vi "Get SMO HELP.vi"(8 "error in (no error)":errorcluster, 10 "Command":string, 11 "Instrument.Lockin in":refnum<class "Instrument.Lockin.lvclass">) -> (0 "error out":errorcluster, 2 "help cluster":T1, 3 "Instrument.Lockin out":refnum<class "Instrument.Lockin.lvclass">)   [LabVIEW 2019, in "Instrument.Lockin.lvlib" / "Instrument.Lockin.lvclass"]
uses:
  Instrument.Lockin.lvclass
  <userlib>/LevyLab/Instrument Framework/subsystems/Help/typedefs/Help--cluster.ctl
  Typedefs/API/Lockin.Commands--Enum.ctl
  Instrument.DAQ/Typedefs/AO.Channel--Cluster.ctl
  Instrument.DAQ/Typedefs/AO.Channel.Function--Enum.ctl
  Instrument.DAQ/Typedefs/AO.Channel--Cluster--Array.ctl
  Typedefs/API/Lockin.setAO_Amp--cluster.ctl
  Typedefs/API/Lockin.setAO_DC--cluster.ctl
  Typedefs/API/Lockin.setAO_f--cluster.ctl
  Typedefs/API/Lockin.setAO_phi--cluster.ctl
  Typedefs/API/Lockin.setAO_function--cluster.ctl
  Instrument.DAQ/Typedefs/REF.Channel--Cluster.ctl
  Instrument.DAQ/Typedefs/REF.Channel--Cluster--Array.ctl
  Typedefs/API/Lockin.setREF_f--cluster.ctl
  Typedefs/API/Lockin.setREF_phi--cluster.ctl
  Typedefs/API/Lockin.setREF_TC--cluster.ctl
  Typedefs/API/Lockin.setREF_RollOff--cluster.ctl
  Instrument.DAQ/Typedefs/DAQ.Configuration--Cluster.ctl
  Instrument.DAQ/Typedefs/DAQ.Config.AO.Range--enum.ctl
  Instrument.DAQ/Typedefs/DAQ.TerminalConfiguration--ring.ctl
  Instrument.DAQ/Typedefs/DAQ.Config.AI.Range--enum.ctl
  Instrument.DAQ/Typedefs/DAQ.Config.AI.Coupling--enum.ctl
  Instrument.DAQ/Typedefs/DAQ.Configuration--Cluster--Array.ctl
  <userlib>/LevyLab/Instrument Framework/Instrument Types/Lockin/Typedefs/LockinAPI.Sampling.Sampling--Cluster.ctl
  Typedefs/API/Lockin.setState--cluster.ctl
  Instrument.DAQ/Typedefs/State--enum.ctl
  Instrument.DAQ/Typedefs/Sweep.Configuration--Cluster.ctl
  Instrument.DAQ/Typedefs/Sweep.Channel--Cluster--Array.ctl
  Instrument.DAQ/Typedefs/Sweep.Channel--Cluster.ctl
  Instrument.DAQ/Typedefs/Sweep.Pattern--Enum.ctl
  Typedefs/API/Lockin.setSweep_Time--cluster.ctl
  Typedefs/API/Lockin.setSweep_Table--cluster.ctl
  <userlib>/LevyLab/Instrument Framework/Instrument Types/Lockin/Typedefs/LockinAPI.getState.states--enum.ctl
  Instrument.DAQ/Typedefs/Results--Cluster.ctl
  <userlib>/LevyLab/Instrument Framework/Instrument Types/Lockin/Typedefs/LockinAPI.SweepData--Cluster.ctl
  <userlib>/LevyLab/Instrument Framework/Instrument Types/Lockin/Instrument.LockinAPI.lvclass
  <userlib>/LevyLab/Instrument Framework/Instrument/Typedefs/Instrument.IDN--cluster.ctl
  <userlib>/LevyLab/Instrument Framework/Instrument/Instrument.lvclass
  <vilib>/PRIrvin/JSON-Schema/JSON-Schema.lvlib
  Instrument.DAQ/Instrument.DAQ.lvclass
  <userlib>/LevyLab/Instrument Framework/subsystems/Help/Help.lvclass
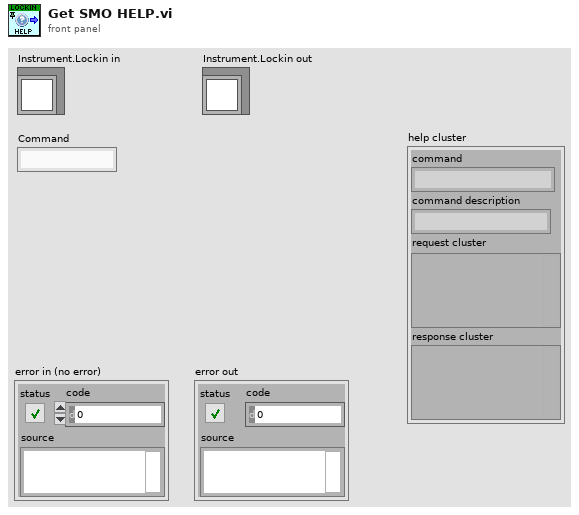
[diagram p1: front panel]
types:
  T1 = typedef "Instrument.lvlib/Help.lvclass/Help--cluster.ctl" = cluster{"command":string, "command description":string, "request cluster":variant, "response cluster":variant}
  T2 = typedef "Instrument.Lockin.lvlib/Instrument.Lockin.lvclass/Lockin.Commands--Enum.ctl" = enum16{"setAO", "setAO_Amplitude", "setAO_DC", "setAO_Frequency", "setAO_Phase", "setAO_Function", "setREF", "setREF_Frequency", "setREF_Phase", "setREF_TC", "setREF_Roll-Off", "setDAQ", "setSampling", "setState", "getState", "getAO", "getAI", "getResults", "getSampling", "getAOconfig", "getREFconfig", "setInputGain", "setOutputGain", "getInputGain", "getOutputGain", "setSweep", "setSweep_Time", "setSweep_Table", "getStatus", "getSweepResults", "getSweepWaveforms", "logConfiguration", "startLogging", "stopLogging"}
  T3 = typedef "Instrument.Lockin.lvlib/Instrument.DAQ.lvclass/AO.Channel--Cluster.ctl" = cluster{"Enable?":bool, "Channel":i32, "Amplitude":dbl, "Offset":dbl, "Frequency":dbl, "Phase":dbl, "Function":T4, "Sweeping?":bool, "Limit AC":bool, "Limit DC?":bool, "Duty Cycle":bool}
  T4 = typedef "Instrument.Lockin.lvlib/Instrument.DAQ.lvclass/AO.Channel.Function--Enum.ctl" = enum16{"sine", "square", "triangle", "saw"}
  T5 = typedef "Instrument.Lockin.lvlib/Instrument.DAQ.lvclass/REF.Channel--Cluster.ctl" = cluster{"Enable?":bool, "Channel":i32, "Frequency":dbl, "Phase":dbl, "TC":dbl, "Roll-Off":i32}
  T6 = typedef "Instrument.Lockin.lvlib/Instrument.DAQ.lvclass/DAQ.Configuration--Cluster.ctl" = cluster{"Device":string, "Lockin.AO":string, "AO.Ch":string, "AO.Range":T7, "AO terminal config":T8, "Lockin.AI":string, "AI.Ch":string, "AI.Range":T9, "AI.Coupling":T10, "AI terminal config":T8}
  T7 = typedef "Instrument.Lockin.lvlib/Instrument.DAQ.lvclass/DAQ.Config.AO.Range--enum.ctl" = enum16{"±0.1", "±1.0", "±3.5", "±10.0", ""}
  T8 = typedef "Instrument.Lockin.lvlib/Instrument.DAQ.lvclass/DAQ.TerminalConfiguration--ring.ctl" = i32
  T9 = typedef "Instrument.Lockin.lvlib/Instrument.DAQ.lvclass/DAQ.Config.AI.Range--enum.ctl" = enum16{"±0.316", "±1.00", "±3.16", "±10.0", "±31.6", "±42.4", ""}
  T10 = typedef "Instrument.Lockin.lvlib/Instrument.DAQ.lvclass/DAQ.Config.AI.Coupling--enum.ctl" = u16
  T11 = typedef "Instrument.Lockin.lvlib/Instrument.Lockin.lvclass/Lockin.setSweep_Table--cluster.ctl" = cluster{"Channel":i32, "Table":dbl[]}
  T12 = typedef "Instrument.LockinAPI.lvclass/LockinAPI.SweepData--Cluster.ctl" = cluster{"AO":waveform(dbl)[], "AI":waveform(dbl)[], "X":waveform(dbl)[], "Y":waveform(dbl)[]}
  T13 = typedef "Instrument.Lockin.lvlib/Instrument.DAQ.lvclass/AO.Channel--Cluster--Array.ctl" = T3[]
  T14 = typedef "Instrument.Lockin.lvlib/Instrument.Lockin.lvclass/Lockin.setAO_Amp--cluster.ctl" = cluster{"Channel":i32, "Amplitude":dbl}
  T15 = typedef "Instrument.Lockin.lvlib/Instrument.Lockin.lvclass/Lockin.setAO_DC--cluster.ctl" = cluster{"Channel":i32, "DC":dbl}
  T16 = typedef "Instrument.Lockin.lvlib/Instrument.Lockin.lvclass/Lockin.setAO_f--cluster.ctl" = cluster{"Channel":i32, "Frequency":dbl}
  T17 = typedef "Instrument.Lockin.lvlib/Instrument.Lockin.lvclass/Lockin.setAO_phi--cluster.ctl" = cluster{"Channel":i32, "Phase":dbl}
  T18 = typedef "Instrument.Lockin.lvlib/Instrument.Lockin.lvclass/Lockin.setAO_function--cluster.ctl" = cluster{"Channel":i32, "Function":T4}
  T19 = typedef "Instrument.Lockin.lvlib/Instrument.DAQ.lvclass/REF.Channel--Cluster--Array.ctl" = T5[]
  T20 = typedef "Instrument.Lockin.lvlib/Instrument.Lockin.lvclass/Lockin.setREF_f--cluster.ctl" = cluster{"Channel":i32, "Frequency":dbl}
  T21 = typedef "Instrument.Lockin.lvlib/Instrument.Lockin.lvclass/Lockin.setREF_phi--cluster.ctl" = cluster{"Channel":i32, "Phase":dbl}
  T22 = typedef "Instrument.Lockin.lvlib/Instrument.Lockin.lvclass/Lockin.setREF_TC--cluster.ctl" = cluster{"Channel":i32, "TC":dbl}
  T23 = typedef "Instrument.Lockin.lvlib/Instrument.Lockin.lvclass/Lockin.setREF_RollOff--cluster.ctl" = cluster{"Channel":i32, "Roll-Off":i32}
  T24 = typedef "Instrument.Lockin.lvlib/Instrument.DAQ.lvclass/DAQ.Configuration--Cluster--Array.ctl" = T6[]
  T25 = typedef "Instrument.LockinAPI.lvclass/LockinAPI.Sampling.Sampling--Cluster.ctl" = cluster{"Fs":dbl, "#s":i32}
  T26 = typedef "Instrument.Lockin.lvlib/Instrument.Lockin.lvclass/Lockin.setState--cluster.ctl" = cluster{"State":T27}
  T27 = typedef "Instrument.Lockin.lvlib/Instrument.DAQ.lvclass/State--enum.ctl" = enum16{"start", "stop", "reset", "start sweep", "stop sweep"}
  T28 = typedef "Instrument.Lockin.lvlib/Instrument.DAQ.lvclass/Sweep.Configuration--Cluster.ctl" = cluster{"sweepTime":dbl, "initialWaitTime":dbl, "returnToStart":bool, "sweepChannels":T29}
  T29 = typedef "Instrument.Lockin.lvlib/Instrument.DAQ.lvclass/Sweep.Channel--Cluster--Array.ctl" = T30[]
  T30 = typedef "Instrument.Lockin.lvlib/Instrument.DAQ.lvclass/Sweep.Channel--Cluster.ctl" = cluster{"Enable?":bool, "Channel":u16, "Start":dbl, "End":dbl, "Pattern":T31, "Table":dbl[]}
  T31 = typedef "Instrument.Lockin.lvlib/Instrument.DAQ.lvclass/Sweep.Pattern--Enum.ctl" = enum16{"Ramp /", "Ramp /\\", "Smooth Ramp _/", "Smooth Ramp _/\\_", "Table"}
  T32 = typedef "Instrument.Lockin.lvlib/Instrument.Lockin.lvclass/Lockin.setSweep_Time--cluster.ctl" = cluster{"SweepTime":dbl}
  T33 = typedef "Instrument.LockinAPI.lvclass/LockinAPI.getState.states--enum.ctl" = enum16{"idle", "created", "started", "stopped", "sweeping"}
  T34 = typedef "Instrument.Lockin.lvlib/Instrument.DAQ.lvclass/Results--Cluster.ctl" = cluster{"Time Stamp":timestamp, "Results (Dictionary)":cluster{"key":string, "value":dbl[]}[]}
  T35 = typedef "Instrument.lvlib/Instrument.lvclass/Instrument.IDN--cluster.ctl" = cluster{"vendor":string, "model":string, "serial":string, "firmware":string}
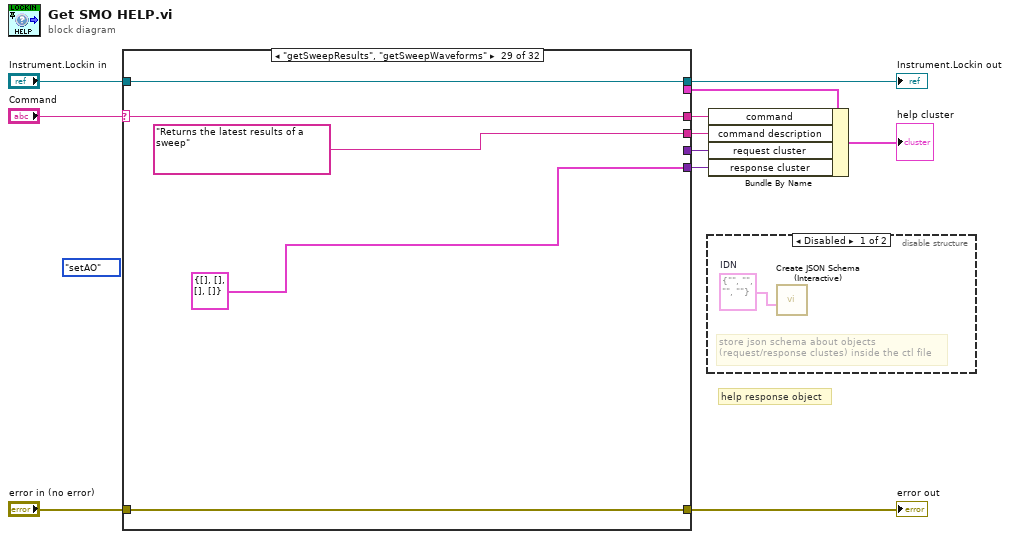
[diagram p0: block diagram]
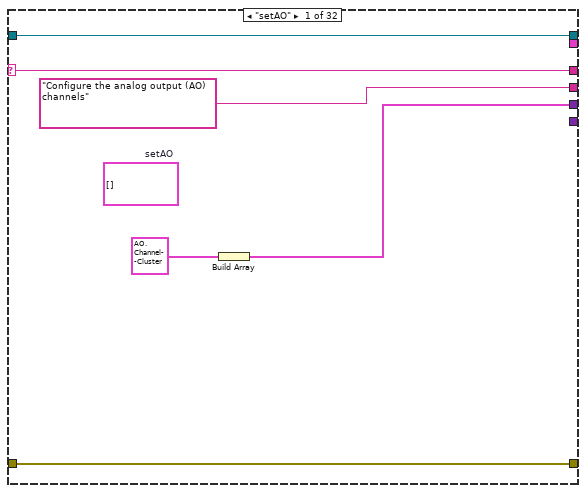
[diagram p2: hidden frame]
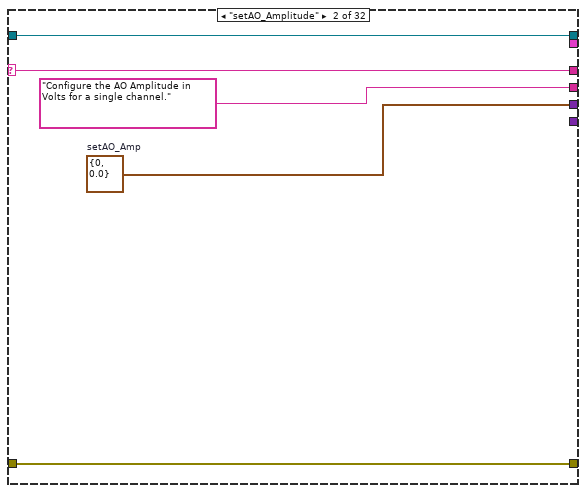
[diagram p3: hidden frame]
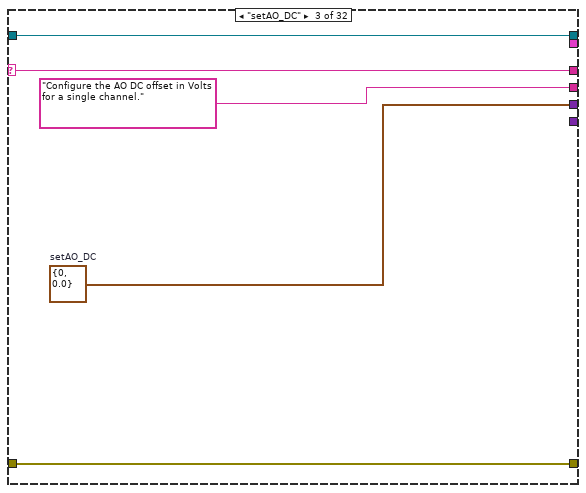
[diagram p4: hidden frame]
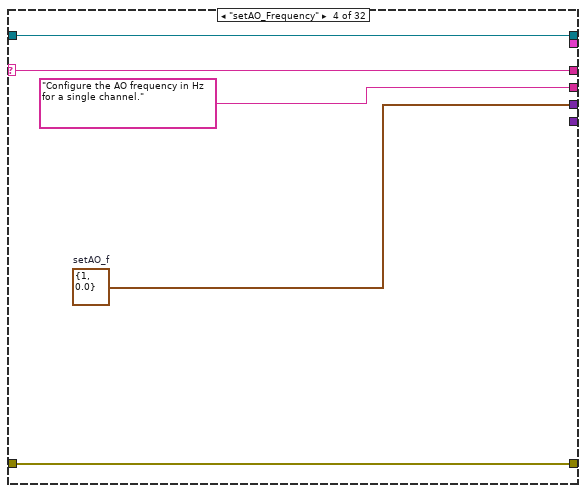
[diagram p5: hidden frame]
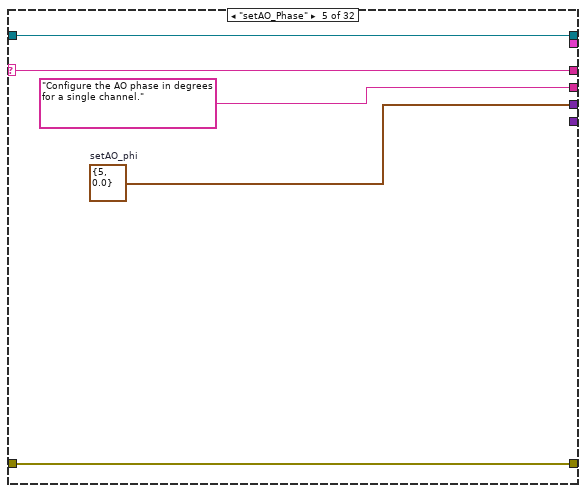
[diagram p6: hidden frame]
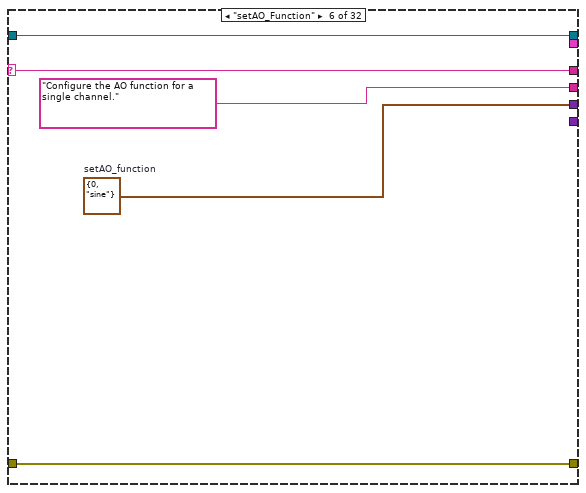
[diagram p7: hidden frame]
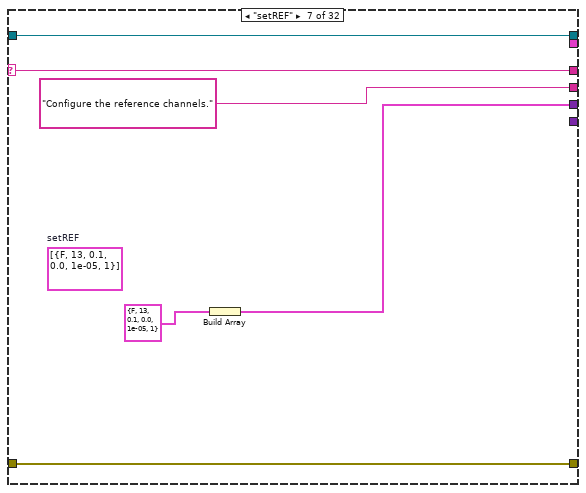
[diagram p8: hidden frame]
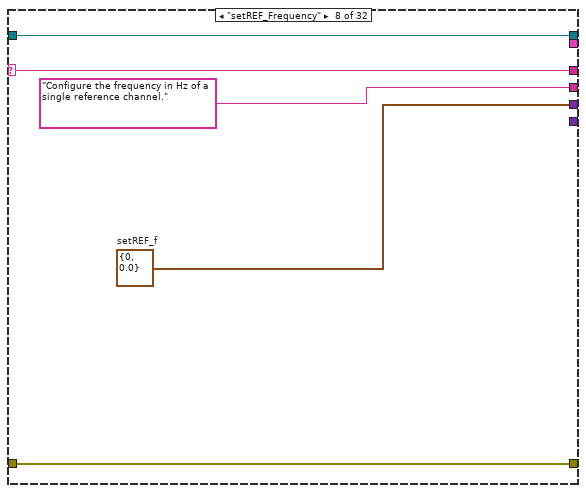
[diagram p9: hidden frame]
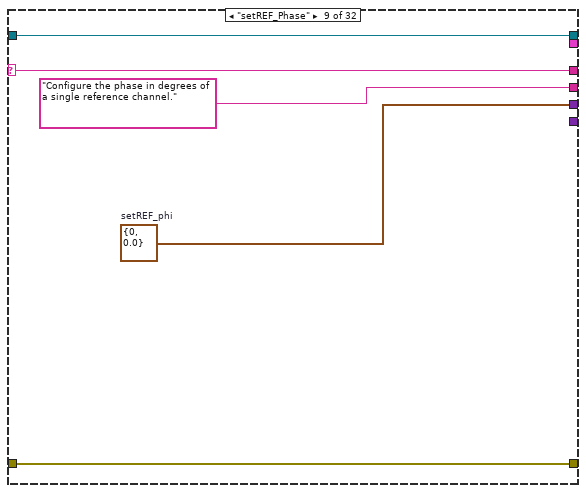
[diagram p10: hidden frame]
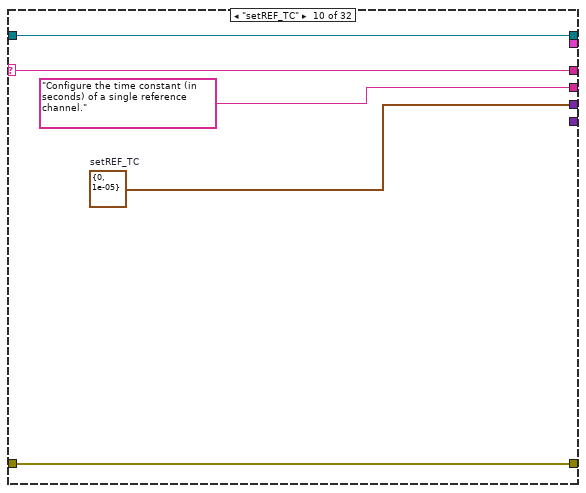
[diagram p11: hidden frame]
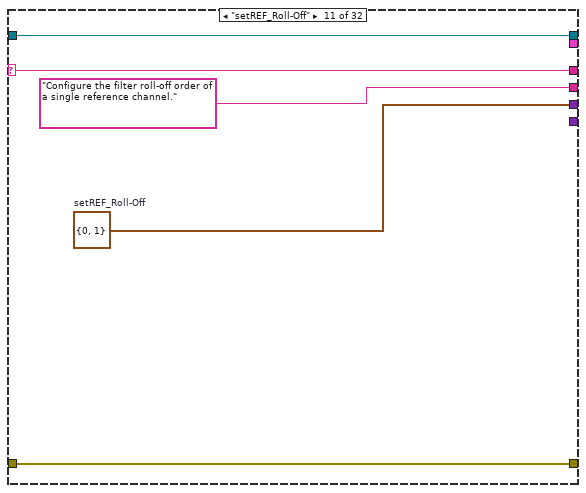
[diagram p12: hidden frame]
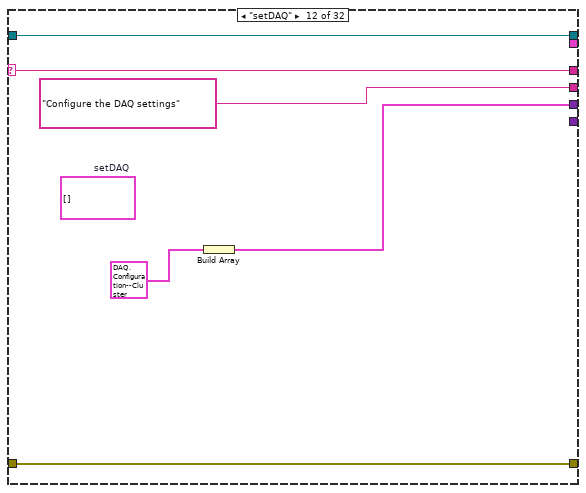
[diagram p13: hidden frame]
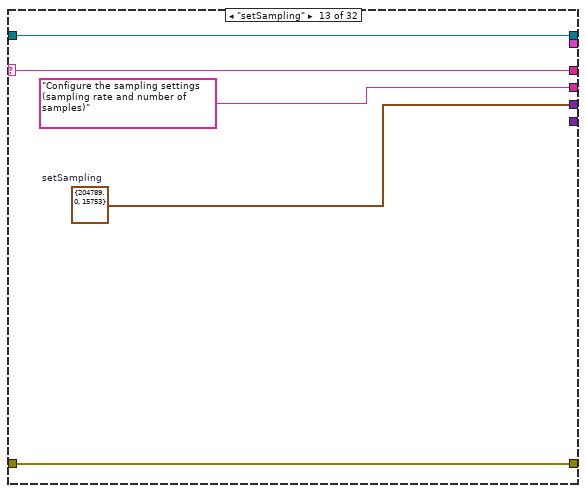
[diagram p14: hidden frame]
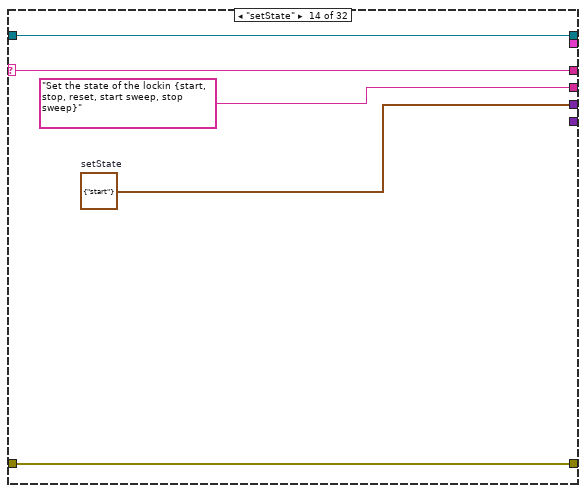
[diagram p15: hidden frame]
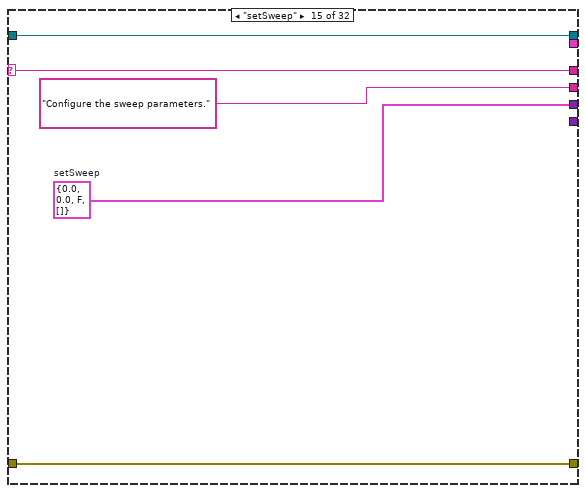
[diagram p16: hidden frame]
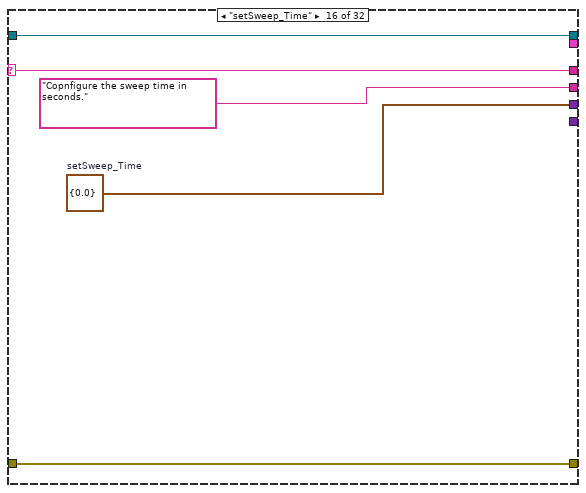
[diagram p17: hidden frame]
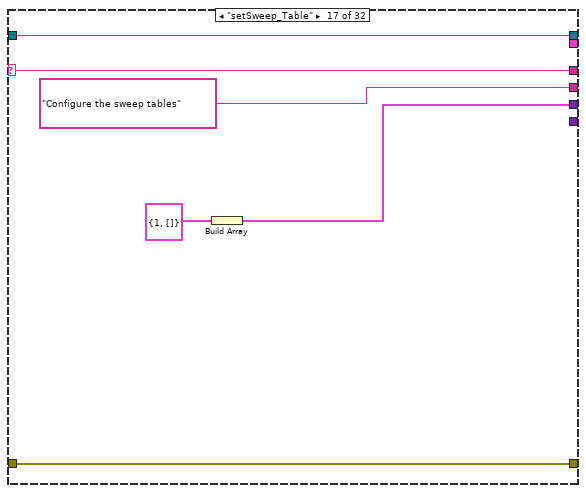
[diagram p18: hidden frame]
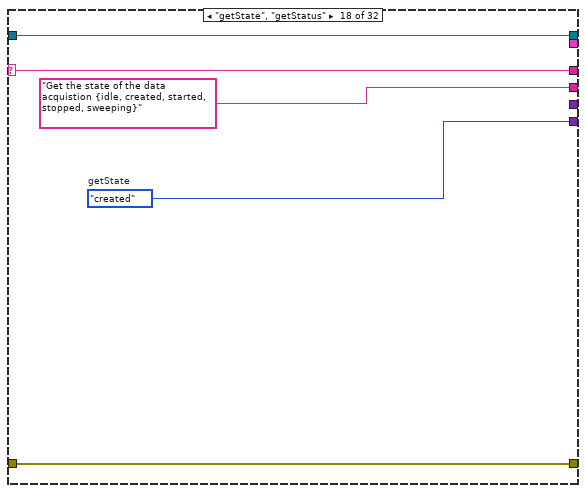
[diagram p19: hidden frame]
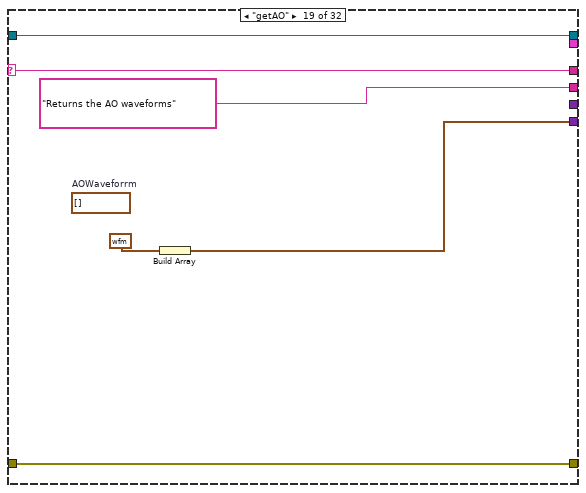
[diagram p20: hidden frame]
diagram:
  (unwired) Lockin.Commands--Enum."setAO" ("Enum")
  # "help response object"
  n1 = case shown="\"getSweepResults\", \"getSweepWaveforms\"" "Command" {
    selector: "Command" -> [w17 w22 w27 w32 w37 w42 w48 w53 w58 w63 w68 w74 w79 w84 w89 w94 w100 w105 w111 w117 w122 w127 w133 w139 w145 w151 w157 w163 w168 w172 w176 w182]
    tunnel: [w17 w22 w27 w32 w37 w42 w48 w53 w58 w63 w68 w74 w79 w84 w89 w94 w100 w105 w111 w117 w122 w127 w133 w139 w145 w151 w157 w163 w168 w172 w176 w183] -> w6
    tunnel: "error in (no error)" -> [w16 w21 w26 w31 w36 w41 w47 w52 w57 w62 w67 w73 w78 w83 w88 w93 w99 w104 w110 w116 w121 w126 w132 w138 w144 w150 w156 w162 w167 w171 w175 w178]
    tunnel: [w16 w21 w26 w31 w36 w41 w47 w52 w57 w62 w67 w73 w78 w83 w88 w93 w99 w104 w110 w116 w121 w126 w132 w138 w144 w150 w156 w162 w167 w171 w175 w177] -> w7
    tunnel: ["Configure the analog output (AO) channels" "Configure the AO Amplitude in Volts for a single channel." "Configure the AO DC offset in Volts for a single channel." "Configure the AO frequency in Hz for a single channel." "Configure the AO phase in degrees for a single channel." "Configure the AO function for a single channel." "Configure the reference channels." "Configure the frequency in Hz of a single reference channel." "Configure the phase in degrees of a single reference channel." "Configure the time constant (in seconds) of a single reference channel." "Configure the filter roll-off order of a single reference channel." "Configure the DAQ settings" "Configure the sampling settings (sampling rate and number of samples)" "Set the state of the lockin {start, stop, reset, start sweep, stop sweep}" "Configure the sweep parameters." "Copnfigure the sweep time in seconds." "Configure the sweep tables" "Get the state of the data acquistion {idle, created, started, stopped, sweeping}" "Returns the AO waveforms" "Returns the AI waveforms" "Returns the results of the lockin calculations." "Returns the sampling settings (Fs in Samples/second and Samples)" "Returns the configuration of the AO channels." "Describe what your command" "Configures the input gain on the AI channels." "Configure the output gain on the AO channels." "Returns the input gain on the AI channels." "Returns the output gain on the AO channels" "Returns the latest results of a sweep" "Start a sweep." "Stop an existing sweep." w184] -> w5
    tunnel: [w12 w18 w23 w28 w33 w38 w43 w49 w54 w59 w64 w69 w75 w80 w85 w90 w95 _ _ _ _ _ _ _ w140 w146 _ _ _ _ _ w185] -> w4
    tunnel: [_ _ _ _ _ _ _ _ _ _ _ _ _ _ _ _ _ w101 w106 w112 w118 w123 w128 w134 _ _ w152 w158 T12 {"AO"=[], "AI"=[], "X"=[], "Y"=[]} ("sweepData") _ _ w186] -> w3
    tunnel: "Instrument.Lockin in" -> [w14 w19 w24 w29 w34 w39 w45 w50 w55 w60 w65 w71 w76 w81 w86 w91 w97 w102 w108 w114 w119 w124 w130 w136 w142 w148 w154 w160 w165 w169 w173 w181]
    tunnel: [w14 w19 w24 w29 w34 w39 w45 w50 w55 w60 w65 w71 w76 w81 w86 w91 w97 w102 w108 w114 w119 w124 w130 w136 w142 w148 w154 w160 w165 w169 w173 w180] -> w10
    tunnel: [_ _ _ _ _ _ _ _ _ _ _ _ _ _ _ _ _ _ _ _ _ _ _ _ _ _ _ _ _ _ _ w179] -> w2
    frame "setAO" {
      (unwired) T13 []  # setAO
      n2 = Build Array(T3 {"Enable?"=FALSE, "Channel"=0, "Amplitude"=0.0, "Offset"=0.0, "Frequency"=0.1, "Phase"=0.0, "Function"=enum."sine", "Sweeping?"=FALSE, "Limit AC"=FALSE, "Limit DC?"=FALSE, "Duty Cycle"=FALSE} ("AO")) -> (w12:T3[])
    }
    frame "setAO_Amplitude" {
      w18 = T14 {"Channel"=0, "Amplitude"=0.0}  # setAO_Amp
    }
    frame "setAO_DC" {
      w23 = T15 {"Channel"=0, "DC"=0.0}  # setAO_DC
    }
    frame "setAO_Frequency" {
      w28 = T16 {"Channel"=1, "Frequency"=0.0}  # setAO_f
    }
    frame "setAO_Phase" {
      w33 = T17 {"Channel"=5, "Phase"=0.0}  # setAO_phi
    }
    frame "setAO_Function" {
      w38 = T18 {"Channel"=0, "Function"=enum."sine"}  # setAO_function
    }
    frame "setREF" {
      (unwired) T19 [{"Enable?"=FALSE, "Channel"=13, "Frequency"=0.1, "Phase"=0.0, "TC"=1e-05, "Roll-Off"=1}]  # setREF
      n3 = Build Array(T5 {"Enable?"=FALSE, "Channel"=13, "Frequency"=0.1, "Phase"=0.0, "TC"=1e-05, "Roll-Off"=1} ("REF")) -> (w43:T5[])
    }
    frame "setREF_Frequency" {
      w49 = T20 {"Channel"=0, "Frequency"=0.0}  # setREF_f
    }
    frame "setREF_Phase" {
      w54 = T21 {"Channel"=0, "Phase"=0.0}  # setREF_phi
    }
    frame "setREF_TC" {
      w59 = T22 {"Channel"=0, "TC"=1e-05}  # setREF_TC
    }
    frame "setREF_Roll-Off" {
      w64 = T23 {"Channel"=0, "Roll-Off"=1}  # setREF_Roll-Off
    }
    frame "setDAQ" {
      (unwired) T24 []  # setDAQ
      n4 = Build Array(T6 {"Device"="", "Lockin.AO"="", "AO.Ch"="", "AO.Range"=enum."±0.1", "AO terminal config"=0, "Lockin.AI"="", "AI.Ch"="", "AI.Range"=enum."±0.316", "AI.Coupling"=10050, "AI terminal config"=0} ("System Cluster")) -> (w69:T6[])
    }
    frame "setSampling" {
      w75 = T25 {"Fs"=204789.0, "#s"=15753}  # setSampling
    }
    frame "setState" {
      w80 = T26 {"State"=enum."start"}  # setState
    }
    frame "setSweep" {
      w85 = T28 {"sweepTime"=0.0, "initialWaitTime"=0.0, "returnToStart"=FALSE, "sweepChannels"=[]}  # setSweep
    }
    frame "setSweep_Time" {
      w90 = T32 {"SweepTime"=0.0}  # setSweep_Time
    }
    frame "setSweep_Table" {
      n5 = Build Array(T11 {"Channel"=1, "Table"=[]} ("setSweep_Table")) -> (w95:T11[])
    }
    frame "getState", "getStatus" {
      w101 = LockinAPI.getState.states--enum."created"  # getState
    }
    frame "getAO" {
      (unwired) waveform(dbl)[] []  # AOWaveforrm
      n6 = Build Array(waveform(dbl) {"t0"=timestamp(0 s since 1904-01-01), "dt"=1.0, "Y"=[]} ("Waveform")) -> (w106:waveform(dbl)[])
    }
    frame "getAI" {
      (unwired) waveform(dbl)[] []  # AIWaveform
      n7 = Build Array(waveform(dbl) {"t0"=timestamp(0 s since 1904-01-01), "dt"=1.0, "Y"=[]} ("Waveform")) -> (w112:waveform(dbl)[])
    }
    frame "getResults" {
      w118 = T34 {"Time Stamp"=timestamp(0 s since 1904-01-01), "Results (Dictionary)"=[]}  # Results
    }
    frame "getSampling" {
      w123 = T25 {"Fs"=204789.0, "#s"=15753}  # getSampling
    }
    frame "getAOconfig" {
      (unwired) T13 []  # AOconfig
      n8 = Build Array(T3 {"Enable?"=FALSE, "Channel"=0, "Amplitude"=0.0, "Offset"=0.0, "Frequency"=0.1, "Phase"=0.0, "Function"=enum."sine", "Sweeping?"=FALSE, "Limit AC"=FALSE, "Limit DC?"=FALSE, "Duty Cycle"=FALSE} ("AO")) -> (w128:T3[])
    }
    frame "getREFconfig" {
      (unwired) T19 [{"Enable?"=FALSE, "Channel"=13, "Frequency"=0.1, "Phase"=0.0, "TC"=1e-05, "Roll-Off"=1}]  # REFconfig
      n9 = Build Array(T5 {"Enable?"=FALSE, "Channel"=13, "Frequency"=0.1, "Phase"=0.0, "TC"=1e-05, "Roll-Off"=1} ("REF")) -> (w134:T5[])
    }
    frame "setInputGain" {
      (unwired) dbl[] []  # InputGain
      n10 = Build Array(0.0 ("Numeric")) -> (w140:dbl[])
    }
    frame "setOutputGain" {
      (unwired) dbl[] []  # OutputGain
      n11 = Build Array(0.0 ("Numeric")) -> (w146:dbl[])
    }
    frame "getInputGain" {
      (unwired) dbl[] []  # InputGain
      n12 = Build Array(0.0 ("Numeric")) -> (w152:dbl[])
    }
    frame "getOutputGain" {
      (unwired) dbl[] []  # OutputGain
      n13 = Build Array(0.0 ("Numeric")) -> (w158:dbl[])
    }
    frame "getSweepResults", "getSweepWaveforms" {
    }
    frame "startSweep" {
    }
    frame "stopSweep" {
    }
    frame Default {
      # "Replace this Get GMO HELP.vi node with \"Call Parent Method\"\nwhen using this design pattern in override"
      n14 = call-parent "Get SMO HELP.vi"("error in (no error)"=w178, "Command"=w182, "Instrument in"=w181) -> ("error out"=w177:errorcluster, "help cluster"=w179:T1, "Instrument out"=w180:refnum<class "Instrument.Lockin.lvclass">)  [unwired: 6 in]
      n15 = Unbundle By Name(w179) -> ("command"=w183:string, "command description"=w184:string, "request cluster"=w185:variant, "response cluster"=w186:variant)
    }
  }
  "Instrument.Lockin out" <- w10
  "error out" <- w7
  n16 = disable-structure shown="Disabled" {
    frame Disabled {
      w187 = T35 {"vendor"="", "model"="", "serial"="", "firmware"=""}  # IDN
      # "store json schema about objects\n(request/response clustes) inside the ctl file"
      n17 = call <vilib>:"Create JSON Schema (Interactive).vi"("LV Object"=w187) -> ()  [unwired: 9 in, 2 out]
    }
    frame Enabled {
    }
  }
  n18 = Bundle By Name(cluster=w2, "command"=w6, "command description"=w5, "request cluster"=w4, "response cluster"=w3) -> (→"help cluster":T1)
